vi "fpga_feedback.vi"(7 "feedback config":T1, 9 "tip guard?":bool, 10 "input":sgl, 11 "output (in)":T2) -> (2 "fb out":sgl, 3 "output (out)":T2)   [LabVIEW 2021]
doc: "Calculate feedback output with PI controller."
uses:
  fpga_dtype_sgl_8ch.ctl
  fpga_feedback_config.ctl
  <vilib>/rvi/Analysis/control/PID/Typedef/niFpgaPID_PIGains.ctl
  <vilib>/rvi/Analysis/control/PID/Typedef/niFpgaPID_OutputRange.ctl
  <vilib>/rvi/Analysis/control/PID/SubVIs/niFpgaPID_PIWrapper.vi
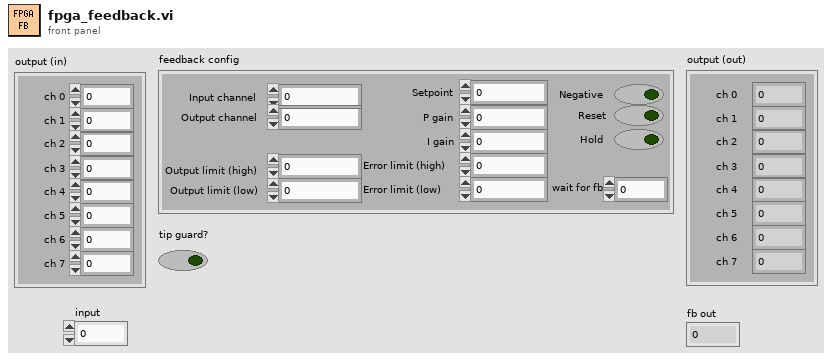
[diagram p1: front panel]
types:
  T1 = typedef "fpga_feedback_config.ctl" = cluster{"Setpoint":sgl, "Output limit (low)":sgl, "Output limit (high)":sgl, "P gain":sgl, "I gain":sgl, "Reset":bool, "Hold":bool, "Negative":bool, "Input channel":i16, "Output channel":i16, "wait for fb":i16, "Error limit (high)":sgl, "Error limit (low)":sgl}
  T2 = typedef "fpga_dtype_sgl_8ch.ctl" = cluster{"ch 0":sgl, "ch 1":sgl, "ch 2":sgl, "ch 3":sgl, "ch 4":sgl, "ch 5":sgl, "ch 6":sgl, "ch 7":sgl}
  T3 = typedef "niFpgaPID_OutputRange.ctl" = cluster{"output high (Inf)":sgl, "output low (-Inf)":sgl}
  T4 = typedef "niFpgaPID_PIGains.ctl" = cluster{"proportional gain":sgl, "integral gain":sgl}
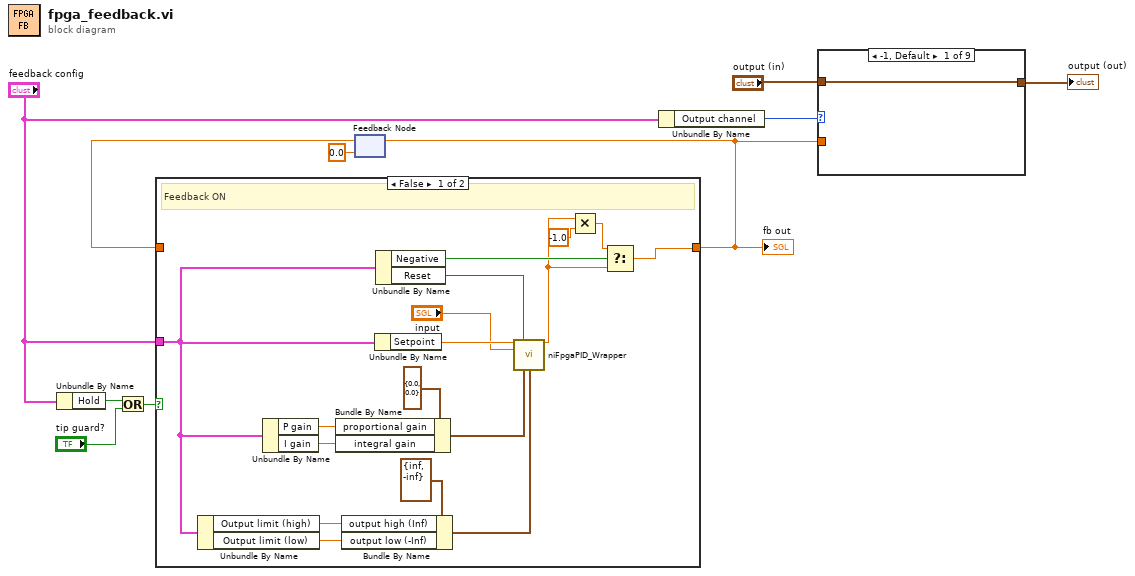
[diagram p0: block diagram]
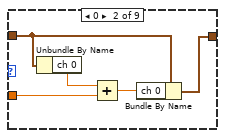
[diagram p2: hidden frame]
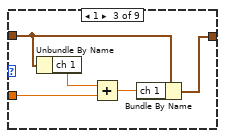
[diagram p3: hidden frame]
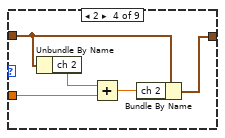
[diagram p4: hidden frame]
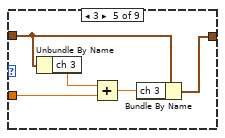
[diagram p5: hidden frame]
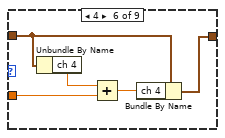
[diagram p6: hidden frame]
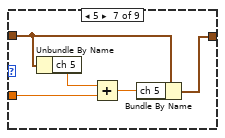
[diagram p7: hidden frame]
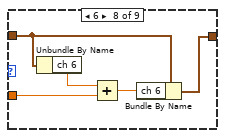
[diagram p8: hidden frame]
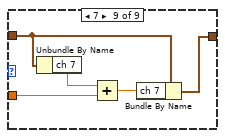
[diagram p9: hidden frame]
diagram:
  n1 = Unbundle By Name("feedback config") -> ("Hold"=w3:bool)
  n2 = Or(x=w3, y="tip guard?") -> (x .or. y?=w1:bool)
  n3 = feedback #1(sgl 0.0 ("output")) -> (w9:sgl)
  n4 = case shown="False" w1 {
    tunnel: [w11 w28] -> w6
    tunnel: "feedback config" -> [w17 _]
    tunnel: w9 -> [_ w28]
    frame False {
      # "Feedback ON"
      n5 = Unbundle By Name(w17) -> ("Output limit (high)"=w22:sgl, "Output limit (low)"=w21:sgl)
      n6 = Unbundle By Name(w17) -> ("P gain"=w26:sgl, "I gain"=w25:sgl)
      n7 = Bundle By Name(cluster=T4 {"proportional gain"=0.0, "integral gain"=0.0} ("gains"), "proportional gain"=w26, "integral gain"=w25) -> (w24:T4)
      n8 = Bundle By Name(cluster=T3 {"output high (Inf)"=inf, "output low (-Inf)"=-inf} ("output range"), "output high (Inf)"=w22, "output low (-Inf)"=w21) -> (w20:T3)
      n9 = Unbundle By Name(w17) -> ("Setpoint"=w19:sgl)
      n10 = Unbundle By Name(w17) -> ("Negative"=w13:bool, "Reset"=w16:bool)
      n11 = call-poly <vilib>:"niFpgaPID_Wrapper.vi"("setpoint"=w19, "reset? (F)"=w16, "process variable"="input", "gains"=w24, "output range"=w20) -> ("output"=w12:sgl)  [unwired: 8 in, 2 out]
      n12 = Multiply(x=w12, y=sgl -1.0) -> (x*y=w14:sgl)
      n13 = Select(t=w14, s=w13, f=w12) -> (s? t:f=w11:sgl)
    }
    frame True {
      # "Feedback Hold"
    }
  }
  "fb out" <- w6
  n14 = feedback-in #1(w6) -> ()
  n15 = Unbundle By Name("feedback config") -> ("Output channel"=w7:i16)
  n16 = case shown="-1, Default" w7 {
    tunnel: w6 -> [_ w32 w37 w42 w47 w52 w57 w62 w67]
    tunnel: "output (in)" -> [w29 w34 w39 w44 w49 w54 w59 w64 w69]
    tunnel: [w29 w30 w35 w40 w45 w50 w55 w60 w65] -> w4
    frame -1, Default {
    }
    frame 0 {
      n17 = Unbundle By Name(w34) -> ("ch 0"=w33:sgl)
      n18 = Add(x=w33, y=w32) -> (x+y=w31:sgl)
      n19 = Bundle By Name(cluster=w34, "ch 0"=w31) -> (w30:T2)
    }
    frame 1 {
      n20 = Unbundle By Name(w39) -> ("ch 1"=w38:sgl)
      n21 = Add(x=w38, y=w37) -> (x+y=w36:sgl)
      n22 = Bundle By Name(cluster=w39, "ch 1"=w36) -> (w35:T2)
    }
    frame 2 {
      n23 = Unbundle By Name(w44) -> ("ch 2"=w43:sgl)
      n24 = Add(x=w43, y=w42) -> (x+y=w41:sgl)
      n25 = Bundle By Name(cluster=w44, "ch 2"=w41) -> (w40:T2)
    }
    frame 3 {
      n26 = Unbundle By Name(w49) -> ("ch 3"=w48:sgl)
      n27 = Add(x=w48, y=w47) -> (x+y=w46:sgl)
      n28 = Bundle By Name(cluster=w49, "ch 3"=w46) -> (w45:T2)
    }
    frame 4 {
      n29 = Unbundle By Name(w54) -> ("ch 4"=w53:sgl)
      n30 = Add(x=w53, y=w52) -> (x+y=w51:sgl)
      n31 = Bundle By Name(cluster=w54, "ch 4"=w51) -> (w50:T2)
    }
    frame 5 {
      n32 = Unbundle By Name(w59) -> ("ch 5"=w58:sgl)
      n33 = Add(x=w58, y=w57) -> (x+y=w56:sgl)
      n34 = Bundle By Name(cluster=w59, "ch 5"=w56) -> (w55:T2)
    }
    frame 6 {
      n35 = Unbundle By Name(w64) -> ("ch 6"=w63:sgl)
      n36 = Add(x=w63, y=w62) -> (x+y=w61:sgl)
      n37 = Bundle By Name(cluster=w64, "ch 6"=w61) -> (w60:T2)
    }
    frame 7 {
      n38 = Unbundle By Name(w69) -> ("ch 7"=w68:sgl)
      n39 = Add(x=w68, y=w67) -> (x+y=w66:sgl)
      n40 = Bundle By Name(cluster=w69, "ch 7"=w66) -> (w65:T2)
    }
  }
  "output (out)" <- w4
